vi "LoadNISTWfrmPluginRequest.vi"(8 "ErrorArray In":errorcluster[](array[cluster]), 10 "clFrontPanelControlRefs":T1) -> (0 "ErrorArray Out":errorcluster[](array[cluster]))   [LabVIEW 2014, in "TestFramework.lvlib"]
uses:
  TestFramework.lvlib
  TypeDefs/clFrontPanelControlRefs.ctl
  FGenPlugins/MyPluginBaseClass/TypeDef/PluginParams.ctl
  WfrmGenerator/WfrmPlugins/EventPluginBaseClass/TypeDefs/dblEvtSignalArray.ctl
  FGenPlugins/MyPluginBaseClass/TypeDef/CreateArbWfrmParams.ctl
  WfrmGenerator/WfrmPlugins/EventPluginBaseClass/TypeDefs/clEvtConfig.ctl
  WfrmGenerator/WfrmModule/PublicAPI/Arguments/Requests/dblEvtParams.ctl
  FGenPlugins/MyPluginBaseClass/TypeDef/ConfigArbWfrmParams.ctl
  FGenPlugins/MyPluginBaseClass/TypeDef/TriggerParams.ctl
  Bus/Public/TypeDefs/clBusData.ctl
  FGenPlugins/MyPluginBaseClass/NISTFGenPluginsBase.lvclass
  Bus/NISTBus.lvclass
  WfrmGenerator/WfrmPlugins/EventPluginBaseClass/BaseWfrmPlugin.lvclass
  WfrmGenerator/WfrmModule/WfrmModule.lvlib
panel:
  # "When you add a control \non the front panel, add a\nreference for it in this\ntype def.  This cluster\nwill hold all of the refer-\nences to the front panel\ncontrols in order to pass\nthese control references \nto subvis."
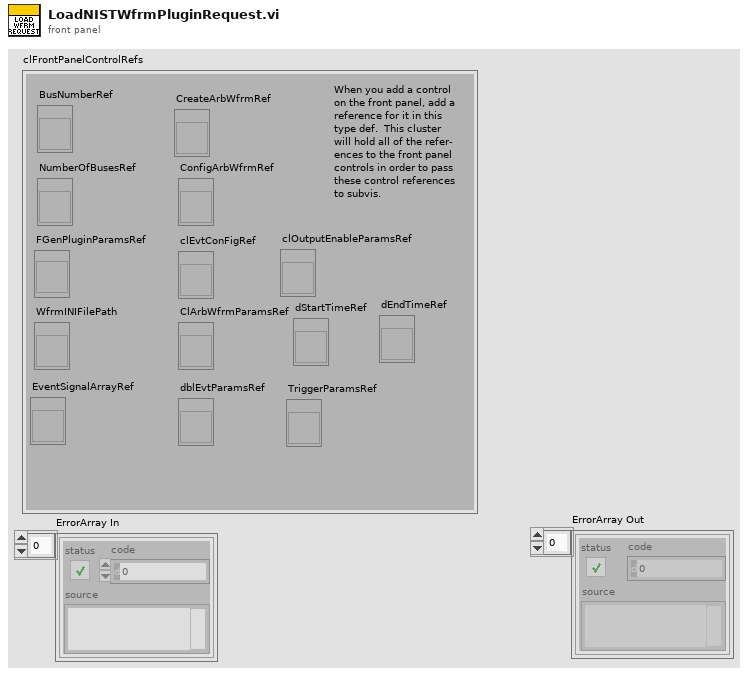
[diagram p1: front panel]
types:
  T1 = typedef "TestFramework.lvlib/clFrontPanelControlRefs.ctl" = cluster{"BusNumberRef":refnum<vi>, "NumberOfBusesRef":refnum<vi>, "FGenPluginParamsRef":refnum<vi>, "WfrmINIFilePath":refnum<vi>, "EventSignalArrayRef":refnum<vi>, "CreateArbWfrmRef":refnum<vi>, "clEvtConFigRef":refnum<vi>, "dblEvtParamsRef":refnum<vi>, "clOutputEnableParamsRef":refnum<vi>, "ConfigArbWfrmRef":refnum<vi>, "ClArbWfrmParamsRef":refnum<vi>, "dStartTimeRef":refnum<vi>, "dEndTimeRef":refnum<vi>, "TriggerParamsRef":refnum<vi>}
  T2 = typedef "Bus.lvlib/NISTBus.lvclass/clBusData.ctl" = cluster{"BusNumber":u8, "NISTWfrmINIFilePath":path, "dblEventSignalArray":dbl[][], "NISTFGenPluginParams":T3}
  T3 = typedef "FGenPlugins.lvlib/NISTFGenPluginsBase.lvclass/PluginParams.ctl" = cluster{"Path to Plugin INI":path}
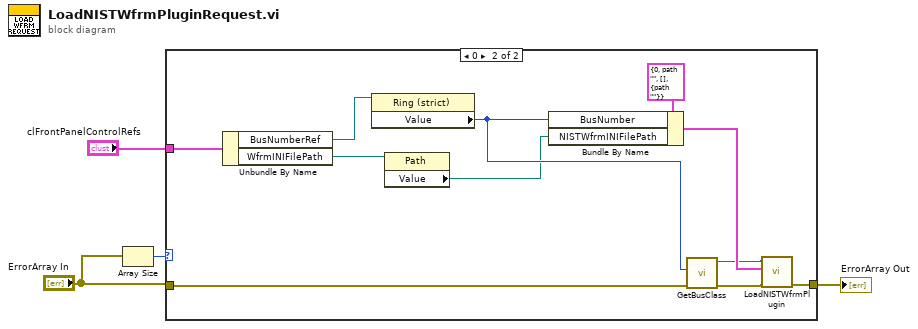
[diagram p0: block diagram]
diagram:
  n1 = Array Size(array="ErrorArray In") -> (size(s)=w3:i32)
  n2 = case shown="0" w3 {
    tunnel: "ErrorArray In" -> [w5 w12]
    tunnel: [w5 w9] -> w1
    tunnel: "clFrontPanelControlRefs" -> [_ w16]
    frame 1, Default {
    }
    frame 0 {
      n3 = Unbundle By Name(w16) -> ("BusNumberRef"=w15:refnum<vi>, "WfrmINIFilePath"=w13:refnum<vi>)
      n4 = property class="Ring (strict)"(reference=w15) -> ("Value"=w11:u8)  [unwired: 1 in, 2 out]
      n5 = property class="Path"(reference=w13) -> ("Value"=w10:path)  [unwired: 1 in, 2 out]
      n6 = Bundle By Name(cluster=T2 {"BusNumber"=0, "NISTWfrmINIFilePath"=path "", "dblEventSignalArray"=[], "NISTFGenPluginParams"={"Path to Plugin INI"=path ""}} ("clBusData"), "BusNumber"=w11, "NISTWfrmINIFilePath"=w10) -> (w7:T2)
      n7 = call "GetBusClass.vi"("ErrorArray In"=w12, "BusNumber"=w11) -> ("ErrorArray Out"=w8:errorcluster[], "NISTBus Out"=w6:refnum<class "NISTBus.lvclass">)  [unwired: 8 in]
      n8 = call "LoadNISTWfrmPlugin.vi"("ErrorArray In"=w8, "clBusData In"=w7, "NISTBus In"=w6) -> ("ErrorArray Out"=w9:errorcluster[])  [unwired: 6 in, 2 out]
    }
  }
  "ErrorArray Out" <- w1
